vi "REPORT_OKNOK_save_csv.vi"(8 "error_in":errorcluster) -> (0 "error_out":errorcluster)   [LabVIEW 2019]
uses:
  FGV/REPORTS_records_display/FGV_REPORTS_records_display.ctl
  typedef/REPORT_OKNOK_all_info.ctl
  _misc/AULocalize/SubVIs/Get Localized Phrase Compact Interface 0D.vi
  <vilib>/Utility/file.llb/Write Delimited Spreadsheet (string).vi
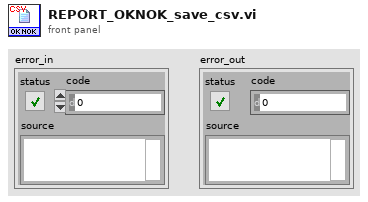
[diagram p1: front panel]
types:
  T1 = typedef "REPORT_OKNOK_all_info.ctl" = cluster{"date_start":string, "date_end":string, "time_start":string, "time_end":string, "records":string[][], "column_headers":string[], "column_widths":i16[]}
  T2 = typedef "FGV_REPORTS_records_display.ctl" = enum16{"initialize", "GEAR_set_serial", "GEAR_set_header", "GEAR_set_operations", "GEAR_set_results", "GEAR_set_batches", "GEAR_get_serial", "GEAR_get_operation_IDs", "GEAR_toggle_results", "GEAR_show_all_results", "GEAR_hide_all_results", "GEAR_display", "GEAR_filter", "GEAR_restore", "GEAR_clear", "GEAR_get_all_info", "DATES_set_dates", "DATES_set_gears", "DATES_display", "DATES_filter", "DATES_first_page", "DATES_previous_page", "DATES_next_page", "DATES_last_page", "DATES_restore", "DATES_clear", "DATES_get_all_info", "PBATCH_set_batch_no", "PBATCH_set_gears", "PBATCH_display", "PBATCH_filter", "PBATCH_first_page", "PBATCH_previous_page", "PBATCH_next_page", "PBATCH_last_page", "PBATCH_restore", "PBATCH_clear", "PBATCH_get_all_info", "OPRTN_set_OP", "OPRTN_set_dates", "OPRTN_set_gears", "OPRTN_set_hidden_columns", "OPRTN_display", "OPRTN_filter", "OPRTN_filter_no_page_reset", "OPRTN_first_page", "OPRTN_previous_page", "OPRTN_next_page", "OPRTN_last_page", "OPRTN_restore", "OPRTN_clear", "OPRTN_get_all_info", "CFG_set_type", "CFG_set_dates", "CFG_set_records", "CFG_display", "CFG_filter", "CFG_first_page", "CFG_previous_page", "CFG_next_page", "CFG_last_page", "CFG_restore", "CFG_clear", "CFG_get_all_info", "AUDIT_set_dates", "AUDIT_set_records", "AUDIT_display", "AUDIT_filter", "AUDIT_first_page", "AUDIT_previous_page", "AUDIT_next_page", "AUDIT_last_page", "AUDIT_restore", "AUDIT_clear", "AUDIT_get_all_info", "OKNOK_set_dates", "OKNOK_set_records", "OKNOK_display", "OKNOK_restore", "OKNOK_clear", "OKNOK_get_all_info", "REWORKS_set_dates", "REWORKS_set_from_to", "REWORKS_set_records", "REWORKS_display", "REWORKS_filter", "REWORKS_first_page", "REWORKS_previous_page", "REWORKS_next_page", "REWORKS_last_page", "REWORKS_restore", "REWORKS_clear", "REWORKS_get_all_info", "PACE_set_dates", "PACE_set_limits", "PACE_set_records", "PACE_display", "PACE_restore", "PACE_clear", "PACE_get_all_info", "CBATCH_set_code", "CBATCH_set_records", "CBATCH_display", "CBATCH_filter", "CBATCH_first_page", "CBATCH_previous_page", "CBATCH_next_page", "CBATCH_last_page", "CBATCH_restore", "CBATCH_clear", "CBATCH_get_all_info", "CMPNT_set_serial", "CMPNT_set_records", "CMPNT_display", "CMPNT_first_page", "CMPNT_previous_page", "CMPNT_next_page", "CMPNT_last_page", "CMPNT_restore", "CMPNT_clear", "CMPNT_get_all_info", "clear"}
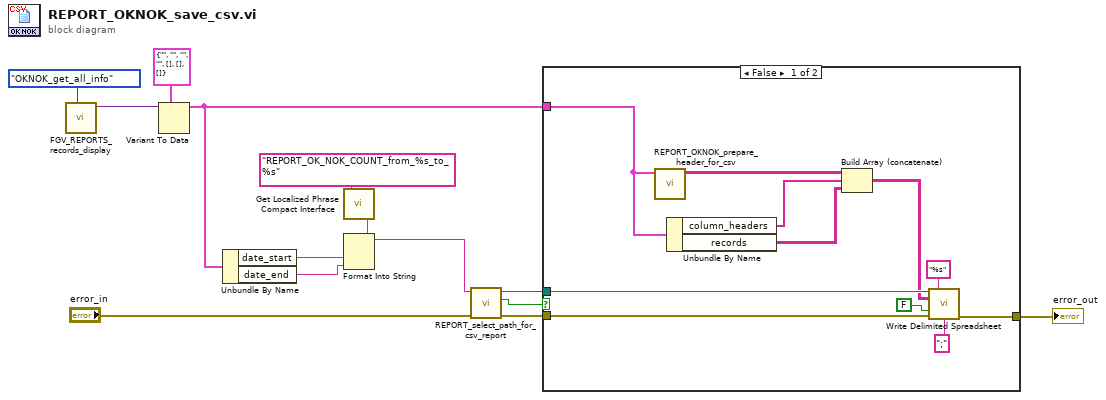
[diagram p0: block diagram]
diagram:
  n1 = call "FGV_REPORTS_records_display.vi"("options"=FGV_REPORTS_records_display."OKNOK_get_all_info") -> ("output"=w14:variant)  [unwired: 9 in, 1 out]
  n2 = Variant To Data(type=T1 {"date_start"="", "date_end"="", "time_start"="", "time_end"="", "records"=[], "column_headers"=[], "column_widths"=[]} ("REPORT_OKNOK_all_info"), Variant=w14) -> (data=w3:T1)  [unwired: 1 in, 1 out]
  n3 = Unbundle By Name(w3) -> ("date_start"=w10:string, "date_end"=w9:string)
  n4 = call-poly "Get Localized Phrase Compact Interface.vi"("Key"="REPORT_OK_NOK_COUNT_from_%s_to_%s" ("report_title")) -> ("Translated Phrase"=w1:string)
  n5 = Format Into String(format string=w1, w10, w9) -> (resulting string=w7:string)  [unwired: 2 in, 1 out]
  n6 = call "REPORT_select_path_for_csv_report.vi"("error_in"="error_in", "report_title"=w7) -> ("error_out"=w5:errorcluster, "Cancelled?"=w6:bool, "path_to_report"=w11:path)  [unwired: 7 in]
  n7 = case shown="False" w6 {
    tunnel: w11 -> [w24 _]
    tunnel: w5 -> [w17 w26]
    tunnel: [w16 w26] -> w4
    tunnel: w3 -> [w15 _]
    frame False {
      n8 = call "REPORT_OKNOK_prepare_header_for_csv.vi"("REPORT_OKNOK_all_info"=w15) -> ("report_header"=w21:string[][])  [unwired: 10 in]
      n9 = Unbundle By Name(w15) -> ("column_headers"=w19:string[], "records"=w18:string[][])
      n10 = Build Array (concatenate)(w21, w19, w18) -> (w20:string[][])
      n11 = call-poly <vilib>:"Write Delimited Spreadsheet.vi"("file path (dialog if empty)"=w24, "format (%s)"="%s" ("format (%.3f)"), "2D data"=w20, "append to file? (new file:F)"=FALSE, "error in (no error)"=w17, "delimiter (\\t)"=";" ("delimiter (\\t)")) -> ("error out"=w16:errorcluster)  [unwired: 8 in, 1 out]
    }
    frame True {
    }
  }
  "error_out" <- w4
